vi "checkFirstTimestamp.vi"(8 "error in (no error)":errorcluster, 11 "WaveformGenerator in":refnum<class "WaveformGenerator.lvclass">) -> (0 "error out":errorcluster, 2 "IsFirst":bool=TRUE, 3 "WaveformGenerator out":refnum<class "WaveformGenerator.lvclass">)   [LabVIEW 2015, in "WaveformGenerator.lvclass"]
uses:
  WaveformGenerator.lvclass
  WaveformGenerator.lvclass/WaveformGenerator.ctl
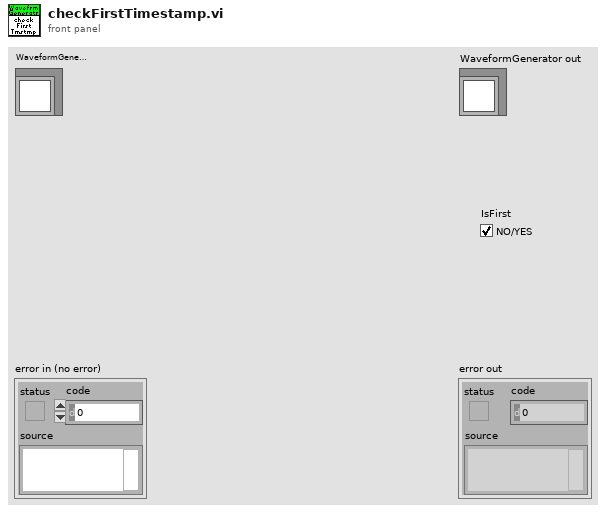
[diagram p1: front panel]
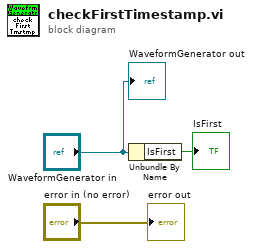
[diagram p0: block diagram]
diagram:
  n1 = Unbundle By Name("WaveformGenerator in") -> ("IsFirst"=→"IsFirst":bool)
  "error out" <- "error in (no error)"
  "WaveformGenerator out" <- "WaveformGenerator in"
